vi "Configure Voltage Source.vi"(0 "VISA resource name":refnum<visa-resource-name>, 1 "Enable LO Connection (F: Disable)":bool, 2 "V-source Range (1.000000E+2)":dbl=100.0 format="%.6e", 5 "Enable V-source (F: Disable)":bool, 7 "Enable Voltage Limit (F: Disable)":bool, 9 "Enable Resistance Current Limit (F: Disable)":bool, 11 "error in (no error)":errorcluster, 12 "Voltage Limit (1.000000E+3)":dbl=1000.0 format="%.6e", 13 "V-source Amplitude (0.000000E+0)":dbl format="%.6e") -> (4 "VISA resource name out":refnum<visa-resource-name>, 15 "error out":errorcluster)   [LabVIEW 2019, in "Keithley 6517.lvlib"]
doc: "Configures V-source settings, enable or disable the V-source, voltage limit, resistance current limit and LO connection, configures the voltage limit, range and amplitude.\n\n<B>Note:</B>\nThis VI is <B>NOT</B> compatible with model <B>6514</B>."
uses:
  Keithley 6517.lvlib
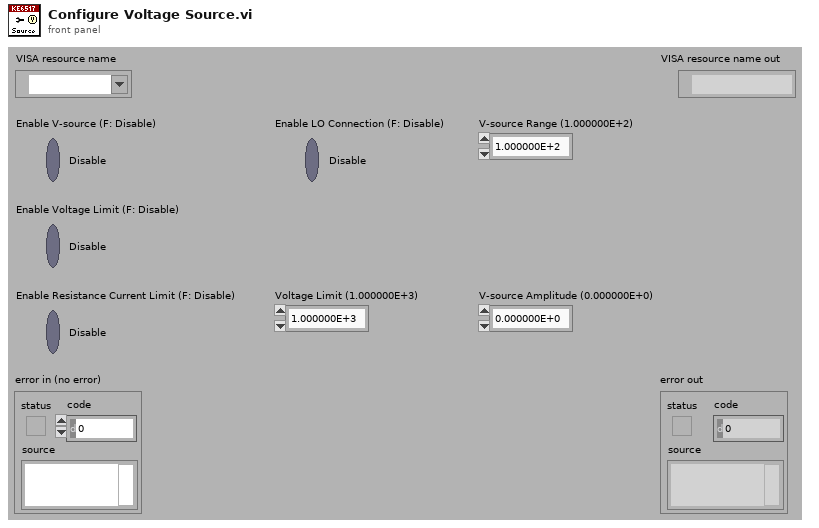
[diagram p1: front panel]
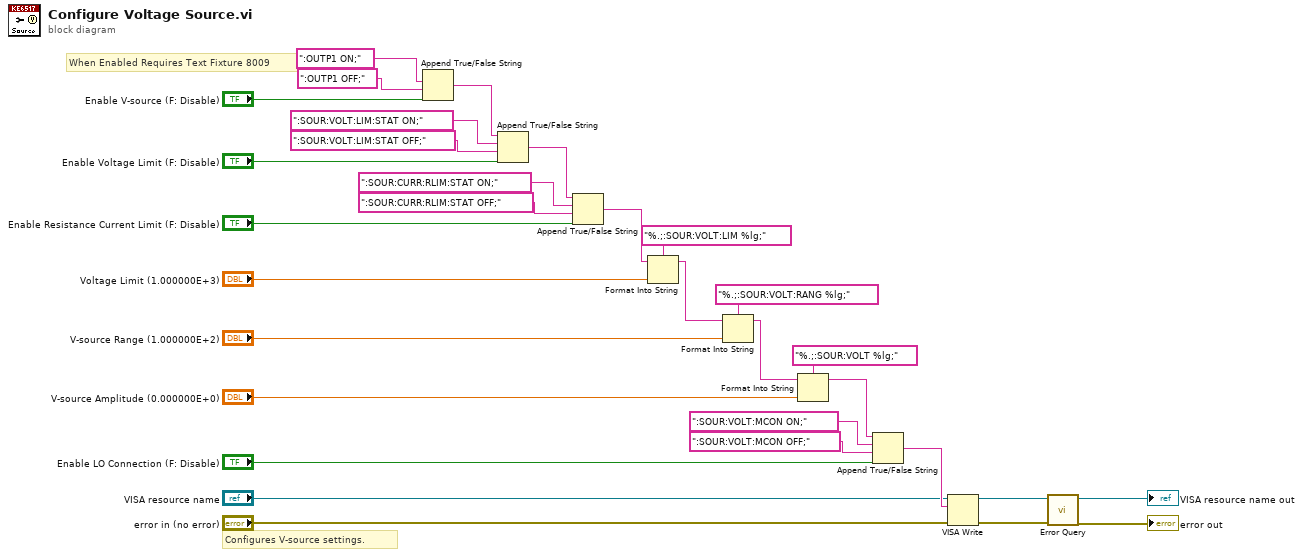
[diagram p0: block diagram]
diagram:
  # "When Enabled Requires Text Fixture 8009"
  # "Configures V-source settings."
  n1 = Append True/False String(1:"Enable V-source (F: Disable)", 2:":OUTP1 OFF;", 3:":OUTP1 ON;") -> (0:w28:string)  [unwired: 1 in]
  n2 = Append True/False String(1:"Enable Voltage Limit (F: Disable)", 2:":SOUR:VOLT:LIM:STAT OFF;", 3:":SOUR:VOLT:LIM:STAT ON;", 4:w28) -> (0:w24:string)
  n3 = Append True/False String(1:"Enable Resistance Current Limit (F: Disable)", 2:":SOUR:CURR:RLIM:STAT OFF;", 3:":SOUR:CURR:RLIM:STAT ON;", 4:w24) -> (0:w20:string)
  n4 = Format Into String(format string="%.;:SOUR:VOLT:LIM %lg;", initial string=w20, "Voltage Limit (1.000000E+3)") -> (resulting string=w17:string)  [unwired: 1 in, 1 out]
  n5 = Format Into String(format string="%.;:SOUR:VOLT:RANG %lg;", initial string=w17, "V-source Range (1.000000E+2)") -> (resulting string=w14:string)  [unwired: 1 in, 1 out]
  n6 = Format Into String(format string="%.;:SOUR:VOLT %lg;", initial string=w14, "V-source Amplitude (0.000000E+0)") -> (resulting string=w11:string)  [unwired: 1 in, 1 out]
  n7 = Append True/False String(1:"Enable LO Connection (F: Disable)", 2:":SOUR:VOLT:MCON OFF;", 3:":SOUR:VOLT:MCON ON;", 4:w11) -> (0:w7:string)
  n8 = VISA Write(VISA resource name="VISA resource name", write buffer=w7, error in (no error)="error in (no error)") -> (VISA resource name out=w4:refnum<visa-resource-name>, error out=w3:errorcluster)  [unwired: 1 out]
  n9 = call "Error Query.vi"("error in (no error)"=w3, "VISA resource name"=w4) -> ("error out"=→"error out":errorcluster, "VISA resource name out"=→"VISA resource name out":refnum<visa-resource-name>)  [unwired: 6 in, 2 out]
